vi "Word_Update_Table.vi"(0 "Word.Tables":refnum<k7>, 1 "Word._Application":refnum<k7>, 5 "value":string[][](array[string]), 7 "table index":i16=-1, 9 "start":cluster{"row":i32, "column":i32}, 11 "error in":errorcluster) -> (15 "error out":errorcluster)   [LabVIEW 2010, in "NI_ReportGenerationToolkit.lvlib"]
uses:
  <vilib>/addons/_office/NI_ReportGenerationToolkit.lvlib
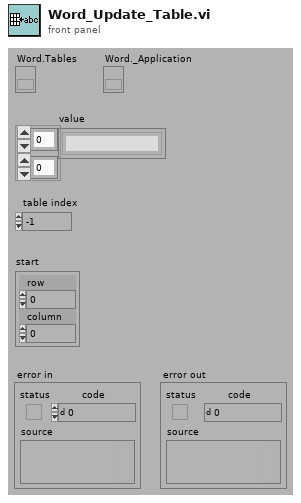
[diagram p1: front panel]
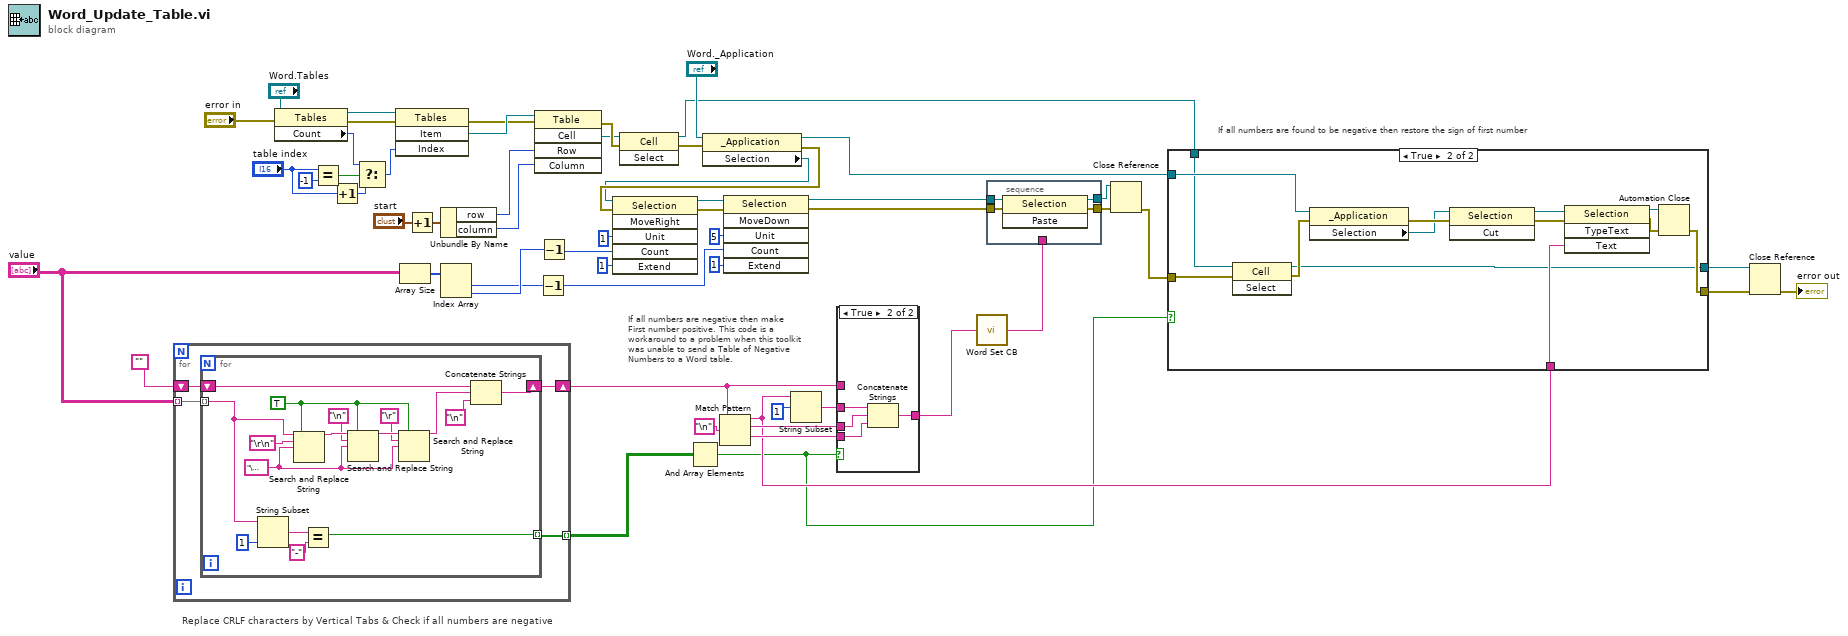
[diagram p0: block diagram]
diagram:
  # "Replace CRLF characters by Vertical Tabs & Check if all numbers are negative"
  # "If all numbers are found to be negative then restore the sign of first number"
  # "If all numbers are negative then make\nFirst number positive. This code is a \nworkaround to a problem when this toolkit\nwas unable to send a Table of Negative \nNumbers to a Word table."
  n1 = for {
    shift-right: [w59] -> w2
    shift-left: "" -> [w60]
    tunnel: "value" -> [w58] mode=indexing
    tunnel: [w57] -> w3 mode=indexing
    n2 = for {
      shift-right: [w75] -> w59
      shift-left: w60 -> [w76]
      tunnel: w58 -> [w65] mode=indexing
      tunnel: [w61] -> w57 mode=indexing
      w66 = TRUE ("replace all? (F)")
      w70 = "\u000b" ("replace string (\"\")")
      n3 = String Subset(string=w65, length (rest)=1 ("length (rest)")) -> (substring=w63:string)  [unwired: 1 out]
      n4 = Search and Replace String(replace all?=w66, input string=w65, search string="\r\n", replace string=w70) -> (result string=w72:string)  [unwired: 1 in, 6 out]
      n5 = Equal?(x=w63, y="-") -> (x = y?=w61:bool)
      n6 = Search and Replace String(replace all?=w66, input string=w72, search string="\n", replace string=w70) -> (result string=w71:string)  [unwired: 1 in, 6 out]
      n7 = Search and Replace String(replace all?=w66, input string=w71, search string="\r", replace string=w70) -> (result string=w69:string)  [unwired: 1 in, 6 out]
      n8 = Concatenate Strings(w76, w69, "\n") -> (w75:string)
    }
  }
  n9 = property class="Tables"(reference="Word.Tables", error in="error in") -> (reference out=w27:refnum<k7>, error out=w25:errorcluster, "Count"=w29:i32)
  n10 = Equal?(x="table index", y=i16 -1) -> (x = y?=w31:bool)
  n11 = Increment(x="table index") -> (x+1=w23:i16)
  n12 = Select(t=w29, s=w31, f=w23) -> (s? t:f=w24:i32)
  n13 = invoke class="Tables" method="Item"(reference=w27, error in=w25, "Index"=w24) -> (error out=w45:errorcluster, "Item"=w52:refnum<k7>)  [unwired: 1 in, 2 out]
  n14 = Array Size(array="value") -> (size(s)=w47:i32[])
  n15 = Increment(x="start") -> (x+1=w20:cluster{"row":i32, "column":i32})
  n16 = Unbundle By Name(w20) -> ("row"=w21:i32, "column"=w22:i32)
  n17 = Index Array(array=w47) -> (element #1=w48:i32, element #2=w49:i32)  [unwired: 2 in]
  n18 = invoke class="Table" method="Cell"(reference=w52, error in=w45, "Row"=w21, "Column"=w22) -> (error out=w35:errorcluster, "Cell"=w34:refnum<k7>)  [unwired: 1 in, 3 out]
  n19 = Decrement(x=w48) -> (x-1=w56:i32)
  n20 = Decrement(x=w49) -> (x-1=w55:i32)
  n21 = invoke class="Cell" method="Select"(reference=w34, error in=w35) -> (reference out=w7:refnum<k7>, error out=w44:errorcluster)  [unwired: 1 in, 1 out]
  n22 = And Array Elements(Boolean array=w3) -> (logical AND=w8:bool)
  n23 = property class="_Application"(reference="Word._Application", error in=w44) -> (reference out=w10:refnum<k7>, error out=w37:errorcluster, "Selection"=w36:refnum<k7>)
  n24 = invoke class="Selection" method="MoveRight"(reference=w36, error in=w37, "Unit"=1, "Count"=w55, "Extend"=1) -> (reference out=w40:refnum<k7>, error out=w41:errorcluster)  [unwired: 1 in, 4 out]
  n25 = Match Pattern(string=w2, regular expression="\n") -> (before substring=w12:string, match substring=w15:string, after substring=w14:string)  [unwired: 2 out]
  n26 = invoke class="Selection" method="MoveDown"(reference=w40, error in=w41, "Unit"=5, "Count"=w56, "Extend"=1) -> (reference out=w50:refnum<k7>, error out=w51:errorcluster)  [unwired: 1 in, 4 out]
  n27 = String Subset(string=w12, offset (0)=1) -> (substring=w17:string)  [unwired: 1 out]
  n28 = case shown="True" w8 {
    tunnel: w2 -> [w77 _]
    tunnel: [w77 w81] -> w13
    tunnel: w17 -> [_ w80]
    tunnel: w15 -> [_ w79]
    tunnel: w14 -> [_ w78]
    frame False {
    }
    frame True {
      n29 = Concatenate Strings(w80, w79, w78) -> (w81:string)
    }
  }
  n30 = call <vilib>:"Word Set CB.vi"("String"=w13) -> ("String 2"=w19:string)
  n31 = stacked-sequence {
    tunnel: w50 -> [w85]
    tunnel: w51 -> [w84]
    tunnel: [w83] -> w53
    tunnel: [w82] -> w54
    tunnel: w19 -> [_]
    frame #0 {
      n32 = invoke class="Selection" method="Paste"(reference=w85, error in=w84) -> (reference out=w82:refnum<k7>, error out=w83:errorcluster)  [unwired: 1 in, 1 out]
    }
  }
  n33 = Close Reference(reference=w54, error in (no error)=w53) -> (error out=w11:errorcluster)
  n34 = case shown="True" w8 {
    tunnel: w11 -> [w87 w89]
    tunnel: w10 -> [_ w97]
    tunnel: [w87 w96] -> w9
    tunnel: w12 -> [_ w95]
    tunnel: w7 -> [w86 w90]
    tunnel: [w86 w88] -> w6
    frame False {
    }
    frame True {
      n35 = invoke class="Cell" method="Select"(reference=w90, error in=w89) -> (reference out=w88:refnum<k7>, error out=w100:errorcluster)  [unwired: 1 in, 1 out]
      n36 = property class="_Application"(reference=w97, error in=w100) -> (error out=w94:errorcluster, "Selection"=w91:refnum<k7>)  [unwired: 1 out]
      n37 = invoke class="Selection" method="Cut"(reference=w91, error in=w94) -> (reference out=w93:refnum<k7>, error out=w92:errorcluster)  [unwired: 1 in, 1 out]
      n38 = invoke class="Selection" method="TypeText"(reference=w93, error in=w92, "Text"=w95) -> (reference out=w98:refnum<k7>, error out=w99:errorcluster)  [unwired: 1 in, 2 out]
      n39 = Automation Close(3:w99, 5:w98) -> (0:w96:errorcluster)
    }
  }
  n40 = Close Reference(reference=w6, error in (no error)=w9) -> (error out=→"error out":errorcluster)
